vi "Create File.vi"(8 "error in":errorcluster, 11 "JSON in":refnum<class "JSON.lvclass">) -> (0 "error out":errorcluster, 3 "JSON out":refnum<class "JSON.lvclass">)   [LabVIEW 2017, in "Report_lib.lvlib" / "JSON.lvclass"]
doc: "This method create or replace\nexternal file for read/write operation"
uses:
  JSON.lvclass
  JSON.lvclass/JSON.ctl
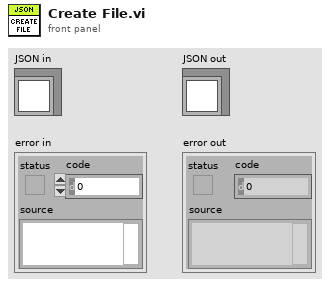
[diagram p1: front panel]
types:
  T1 = enum16{"open", "replace", "create", "open or create", "replace or create", "replace or create with confirmation"}
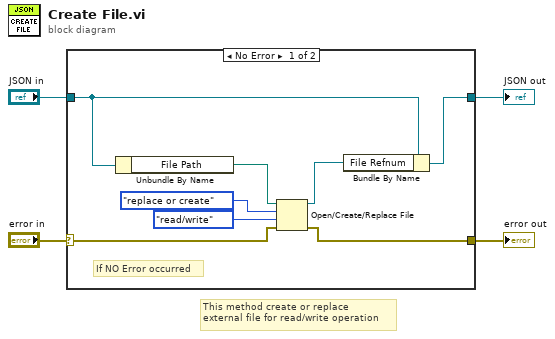
[diagram p0: block diagram]
diagram:
  # "This method create or replace\nexternal file for read/write operation"
  n1 = case shown="No Error" "error in" {
    selector: "error in" -> [w8 w14]
    tunnel: [w7 w14] -> w3
    tunnel: [w6 w13] -> w1
    tunnel: "JSON in" -> [w5 w13]
    frame No Error {
      # "If NO Error occurred"
      n2 = Unbundle By Name(w5) -> ("File Path"=w10:path)
      n3 = Open/Create/Replace File(file path (use dialog)=w10, error in=w8, operation (0:open)=T1."replace or create", access (0:read/write)=enum16{"read/write", "read-only", "write-only"}."read/write") -> (refnum out=w9:refnum<file>, error out=w7:errorcluster)  [unwired: 2 in, 1 out]
      n4 = Bundle By Name(cluster=w5, "File Refnum"=w9) -> (w6:refnum<class "JSON.lvclass">)
    }
    frame Error {
    }
  }
  "error out" <- w3
  "JSON out" <- w1
